vi "SnapImg.vi"(4 "error in (no error)":errorcluster, 7 "session in":refnum<k35>) -> (0 "error out":errorcluster, 2 "img out":T1, 3 "session out":refnum<k35>)   [LabVIEW 2018]
uses:
  <vilib>/picture/picture.llb/imagedata.ctl
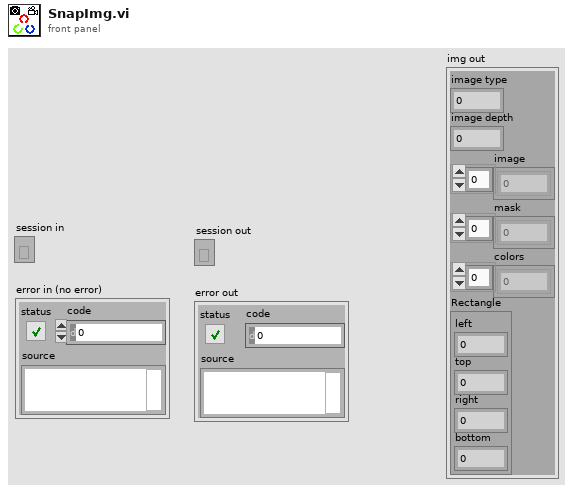
[diagram p1: front panel]
types:
  T1 = typedef "imagedata.ctl" = cluster{"image type":i32, "image depth":i32, "image":u8[], "mask":u8[], "colors":u32[], "Rectangle":cluster{"left":i16, "top":i16, "right":i16, "bottom":i16}}
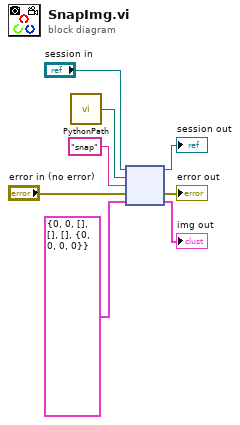
[diagram p0: block diagram]
diagram:
  n1 = call "PythonPath.vi"() -> ("path to .py"=w3:path)
  n2 = node("session in", w3, "snap" ("function name"), "error in (no error)", T1 {"image type"=0, "image depth"=0, "image"=[], "mask"=[], "colors"=[], "Rectangle"={"left"=0, "top"=0, "right"=0, "bottom"=0}} ("image data")) -> (→"session out":refnum<k35>, →"error out":errorcluster, →"img out":T1)  [unwired: 2 out]
